vi "Write Numeric.vi"(8 "error in (no error)":errorcluster, 10 "Numeric":i32, 11 "ConcreteModel in":refnum<class "ConcreteModel.lvclass">) -> (0 "error out":errorcluster, 3 "ConcreteModel out":refnum<class "ConcreteModel.lvclass">)   [LabVIEW 2018, in "TopLevelApplication.lvlib" / "ConcreteModel.lvclass"]
uses:
  ConcreteModel.lvclass
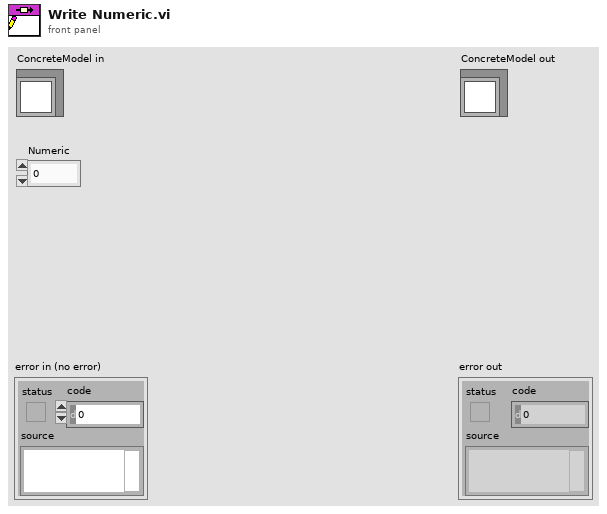
[diagram p1: front panel]
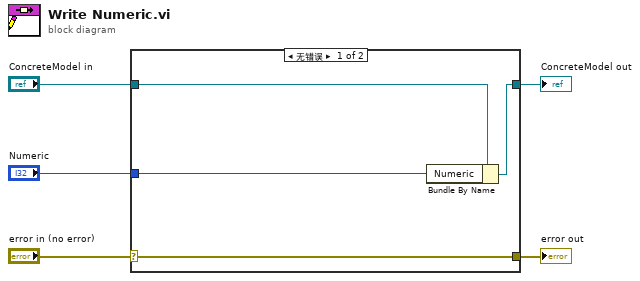
[diagram p0: block diagram]
diagram:
  n1 = case shown="无错误" "error in (no error)" {
    selector: "error in (no error)" -> [w9 w10]
    tunnel: [w9 w10] -> w4
    tunnel: [w7 w11] -> w2
    tunnel: "ConcreteModel in" -> [w8 w11]
    tunnel: "Numeric" -> [w6 _]
    frame No Error {
      n2 = Bundle By Name(cluster=w8, "Numeric"=w6) -> (w7:refnum<class "ConcreteModel.lvclass">)
    }
    frame Error {
    }
  }
  "error out" <- w4
  "ConcreteModel out" <- w2
